vi "Configure Trigger (Window).vi"(0 "VISA resource name":refnum<visa-resource-name>, 1 "Width (5E-10s)":dbl=5e-10, 2 "Upper Level (1.2V)":dbl=1.2, 3 "Lower Level (0.8V)":dbl=0.8, 5 "Source (0:Channel1)":u16(ring) items=["Channel1", "Channel2", "Channel3", "Channel4", "Digital Channel0", "Digital Channel1", "Digital Channel2", "Digital Channel3", "Digital Channel4", "Digital Channel5", "Digital Channel6", "Digital Channel7", "Digital Channel8", "Digital Channel9", "Digital Channel10", "Digital Channel11", "Digital Channel12", "Digital Channel13", "Digital Channel14", "Digital Channel15"], 9 "Trigger Condition(0:Enter Window)":u16(ring) items=["Enter Window", "Exit Window", "Inside > t", "Outside > t"], 11 "error in (no error)":errorcluster, 12 "Trigger If Window (0:Occurs)":u16(ring) items=["Occurs", "Logic"], 13 "Trigger Event (0:A Event)":u16(ring) items=["A Event", "B Event"]) -> (4 "VISA resource name out":refnum<visa-resource-name>, 6 "Trigger Event Out":u16(ring) items=["A Event", "B Event"], 15 "error out":errorcluster)   [LabVIEW 2015, in "Tektronix 7000 Series.lvlib"]
doc: "Configures window trigger settings for an oscilloscope. A window occurs when a pulse meets the <B>Trigger Event</B> conditions.\n\n<B>Note:</B> \nTDS5000,TDS6000,CSA7000 and TDS7000 series oscilloscopes don't support Window Trigger. TDS5000B support A Window Trigger."
uses:
  <instrlib>/Tektronix 7000 Series/Tektronix 7000 Series.lvlib
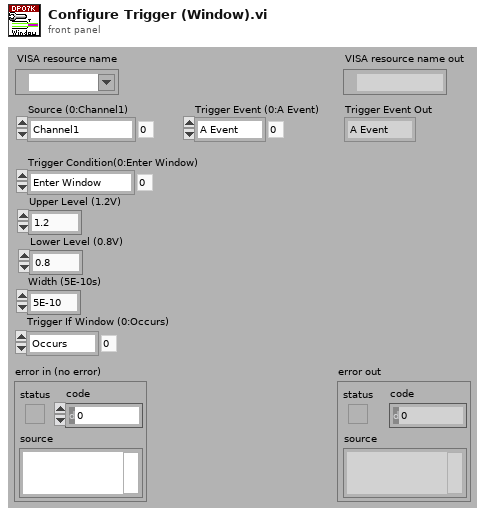
[diagram p1: front panel]
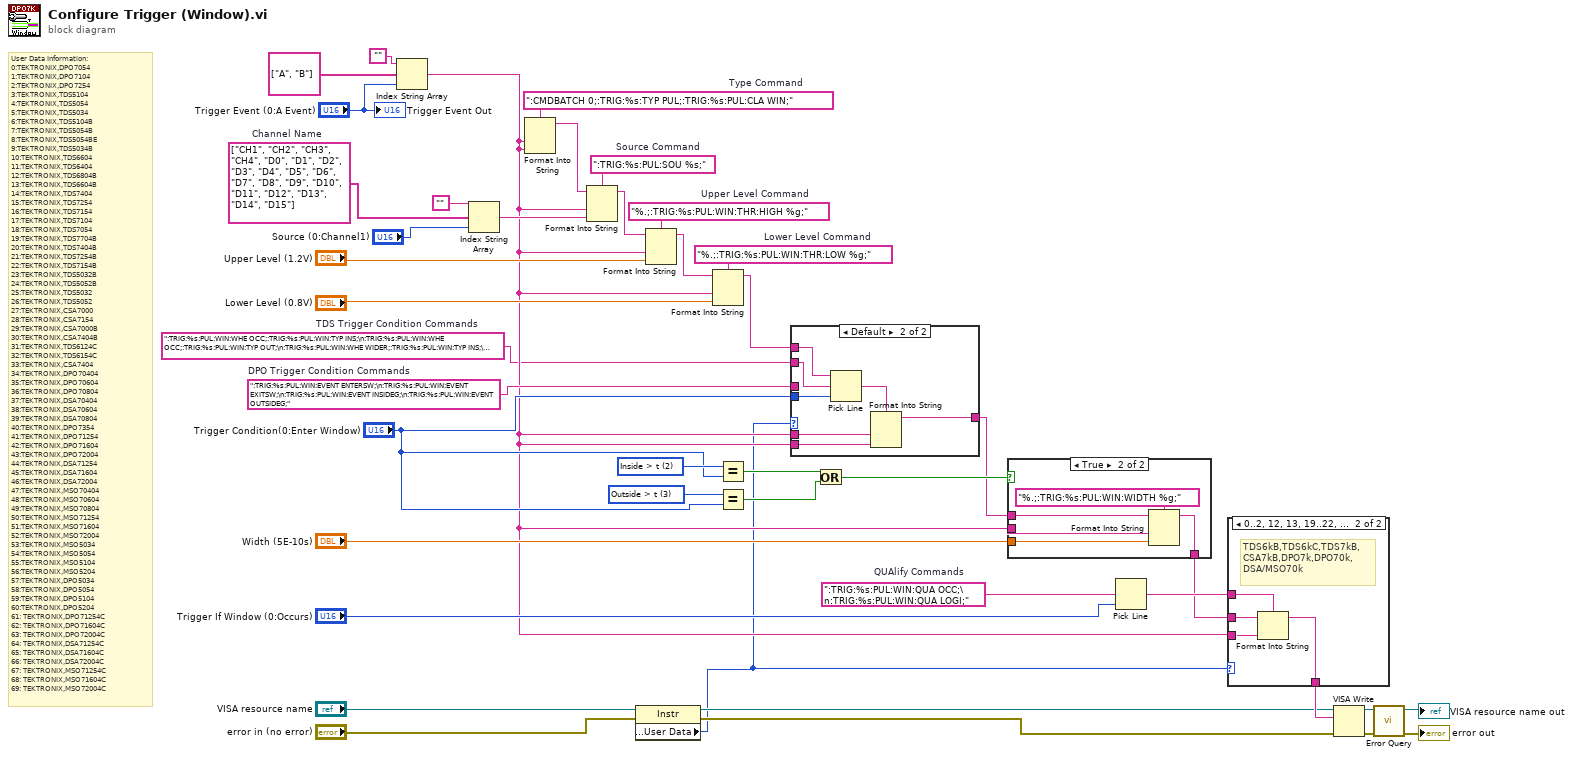
[diagram p0: block diagram]
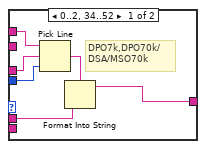
[diagram p2: hidden frame]
diagram:
  w1 = string[] ["CH1", "CH2", "CH3", "CH4", "D0", "D1", "D2", "D3", "D4", "D5", "D6", "D7", "D8", "D9", "D10", "D11", "D12", "D13", "D14", "D15"]  # Channel Name
  w6 = ":TRIG:%s:PUL:WIN:WHE OCC;:TRIG:%s:PUL:WIN:TYP INS;\n:TRIG:%s:PUL:WIN:WHE OCC;:TRIG:%s:PUL:WIN:TYP OUT;\n:TRIG:%s:PUL:WIN:WHE WIDER;:TRIG:%s:PUL:WIN:TYP INS;\n:TRIG:%s:PUL:WIN:WHE WIDER; :TRIG:%s:PUL:WIN:TYP OUT;"  # TDS Trigger Condition Commands
  w23 = ":TRIG:%s:PUL:WIN:QUA OCC;\n:TRIG:%s:PUL:WIN:QUA LOGI;"  # QUAlify Commands
  w25 = "%.;:TRIG:%s:PUL:WIN:THR:HIGH %g;"  # Upper Level Command
  w30 = u16 2 items=["Enter Window", "Exit Window", "Inside > t", "Outside > t"] ("Trigger Condition(0:Enter Window)")
  w29 = u16 3 items=["Enter Window", "Exit Window", "Inside > t", "Outside > t"] ("Trigger Condition(0:Enter Window)")
  w31 = "%.;:TRIG:%s:PUL:WIN:THR:LOW %g;"  # Lower Level Command
  w19 = ":TRIG:%s:PUL:WIN:EVENT ENTERSW;\n:TRIG:%s:PUL:WIN:EVENT EXITSW;\n:TRIG:%s:PUL:WIN:EVENT INSIDEG;\n:TRIG:%s:PUL:WIN:EVENT OUTSIDEG;"  # DPO Trigger Condition Commands
  w32 = ":TRIG:%s:PUL:SOU %s;"  # Source Command
  w22 = ":CMDBATCH 0;:TRIG:%s:TYP PUL;:TRIG:%s:PUL:CLA WIN;"  # Type Command
  # "User Data Information:\n0:TEKTRONIX,DPO7054\n1:TEKTRONIX,DPO7104\n2:TEKTRONIX,DPO7254\n3:TEKTRONIX,TDS5104\n4:TEKTRONIX,TDS5054\n5:TEKTRONIX,TDS5034\n6:TEKTRONIX,TDS5104B\n7:TEKTRONIX,TDS5054B\n8:TEKTRONIX,TDS5054BE\n9:TEKTRONIX,TDS5034B\n10:TEKTRONIX,TDS6604\n11:TEKTRONIX,TDS6404\n12:TEKTRONIX,TDS6804B\n13:TEKTRONIX,TDS6604B\n14:TEKTRONIX,TDS7404\n15:TEKTRONIX,TDS7254\n16:TEKTRONIX,TDS7154\n17:TEKTRONIX,TDS7104\n18:TEKTRONIX,TDS7054\n19:TEKTRONIX,TDS7704B\n20:TEKTRONIX,TDS7404B\n21:TEKTRONIX,TDS7254B\n22:TEKTRONIX,TDS7154B\n23:TEKTRONIX,TDS5032B\n24:TEKTRONIX,TDS5052B\n25:TEKTRONIX,TDS5032\n26:TEKTRONIX,TDS5052\n27:TEKTRONIX,CSA7000\n28:TEKTRONIX,CSA7154\n29:TEKTRONIX,CSA7000B\n30:TEKTRONIX,CSA7404B\n31:TEKTRONIX,TDS6124C\n32:TEKTRONIX,TDS6154C\n33:TEKTRONIX,CSA7404\n34:TEKTRONIX,DPO70404\n35:TEKTRONIX,DPO70604\n36:TEKTRONIX,DPO70804\n37:TEKTRONIX,DSA70404\n38:TEKTRONIX,DSA70604\n39:TEKTRONIX,DSA70804\n40:TEKTRONIX,DPO7354\n41:TEKTRONIX,DPO71254\n42:TEKTRONIX,DPO71604\n43:TEKTRONIX,DPO72004\n44:TEKTRONIX,DSA71254\n45:TEKTRONIX,DSA71604\n46:TEKTRONIX,DSA72004\n47:TEKTRONIX,MSO70404\n48:TEKTRONIX,MSO70604\n49:TEKTRONIX,MSO70804\n50:TEKTRONIX,MSO71254\n51:TEKTRONIX,MSO71604\n52:TEKTRONIX,MSO72004\n53:TEKTRONIX,MSO5034\n54:TEKTRONIX,MSO5054\n55:TEKTRONIX,MSO5104\n56:TEKTRONIX,MSO5204\n57:TEKTRONIX,DPO5034\n58:TEKTRONIX,DPO5054\n59:TEKTRONIX,DPO5104\n60:TEKTRONIX,DPO5204\n61: TEKTRONIX,DPO71254C\n62: TEKTRONIX,DPO71604C\n63: TEKTRONIX,DPO72004C\n64: TEKTRONIX,DSA71254C\n65: TEKTRONIX,DSA71604C\n66: TEKTRONIX,DSA72004C\n67: TEKTRONIX,MSO71254C\n68: TEKTRONIX,MSO71604C\n69: TEKTRONIX,MSO72004C"
  n1 = Index String Array(1:"Trigger Event (0:A Event)", 2:string[] ["A", "B"], 3:"" ("Empty String Constant")) -> (0:w7:string)
  n2 = Index String Array(1:"Source (0:Channel1)", 2:w1, 3:"") -> (0:w20:string)
  n3 = Format Into String(format string=w22, w7, w7) -> (resulting string=w21:string)  [unwired: 2 in, 1 out]
  n4 = Format Into String(format string=w32, initial string=w21, w7, w20) -> (resulting string=w9:string)  [unwired: 1 in, 1 out]
  n5 = property class="Instr"(reference="VISA resource name", error in="error in (no error)") -> (reference out=w12:refnum<visa-resource-name>, error out=w11:errorcluster, "General Settings:User Data"=w3:u32)
  n6 = Format Into String(format string=w25, initial string=w9, w7, "Upper Level (1.2V)") -> (resulting string=w24:string)  [unwired: 1 in, 1 out]
  n7 = Format Into String(format string=w31, initial string=w24, w7, "Lower Level (0.8V)") -> (resulting string=w8:string)  [unwired: 1 in, 1 out]
  n8 = Equal?(x=w30, y="Trigger Condition(0:Enter Window)") -> (x = y?=w28:bool)
  n9 = Equal?(x=w29, y="Trigger Condition(0:Enter Window)") -> (x = y?=w27:bool)
  n10 = case shown="Default" w3 {
    tunnel: w19 -> [w48 _]
    tunnel: "Trigger Condition(0:Enter Window)" -> [w47 w55]
    tunnel: [w45 w53] -> w17
    tunnel: w7 -> [w44 w52]
    tunnel: w8 -> [w43 w51]
    tunnel: w7 -> [_ w50]
    tunnel: w6 -> [_ w49]
    frame 0..2, 34..52 {
      # "DPO7k,DPO70k/\nDSA/MSO70k"
      n11 = Pick Line(string ("")=w43, multi-line string=w48, line index=w47) -> (output string=w46:string)
      n12 = Format Into String(format string=w46, w44) -> (resulting string=w45:string)  [unwired: 2 in, 1 out]
    }
    frame Default {
      n13 = Pick Line(string ("")=w51, multi-line string=w49, line index=w55) -> (output string=w54:string)
      n14 = Format Into String(format string=w54, w52, w50) -> (resulting string=w53:string)  [unwired: 2 in, 1 out]
    }
  }
  n15 = Or(x=w28, y=w27) -> (x .or. y?=w26:bool)
  n16 = case shown="True" w26 {
    tunnel: w17 -> [w56 w60]
    tunnel: [w56 w59] -> w10
    tunnel: "Width (5E-10s)" -> [_ w58]
    tunnel: w7 -> [_ w57]
    frame False {
    }
    frame True {
      n17 = Format Into String(format string="%.;:TRIG:%s:PUL:WIN:WIDTH %g;", initial string=w60, w57, w58) -> (resulting string=w59:string)  [unwired: 1 in, 1 out]
    }
  }
  n18 = Pick Line(multi-line string=w23, line index="Trigger If Window (0:Occurs)") -> (output string=w14:string)  [unwired: 1 in]
  n19 = case shown="0..2, 12, 13, 19..22, 29..32, 34..52, 61..69" w3 {
    tunnel: w14 -> [_ w66]
    tunnel: w7 -> [_ w65]
    tunnel: w10 -> [w62 w64]
    tunnel: [w62 w63] -> w13
    frame Default {
    }
    frame 0..2, 12, 13, 19..22, 29..32, 34..52, 61..69 {
      # "TDS6kB,TDS6kC,TDS7kB,\nCSA7kB,DPO7k,DPO70k, \nDSA/MSO70k"
      n20 = Format Into String(format string=w66, initial string=w64, w65) -> (resulting string=w63:string)  [unwired: 1 in, 1 out]
    }
  }
  n21 = VISA Write(VISA resource name=w12, write buffer=w13, error in (no error)=w11) -> (VISA resource name out=w41:refnum<visa-resource-name>, error out=w40:errorcluster)  [unwired: 1 out]
  n22 = call <instrlib>:"Error Query.vi"("error in (no error)"=w40, "VISA resource name"=w41) -> ("error out"=→"error out":errorcluster, "VISA resource name out"=→"VISA resource name out":refnum<visa-resource-name>)  [unwired: 6 in, 2 out]
  "Trigger Event Out" <- "Trigger Event (0:A Event)"
